vi "SetGet EMIccdGainControlMode.vi"(6 "wait for reply (T)":bool=TRUE, 7 "Broadcast":bool, 8 "error in (no error)":errorcluster, 9 "SetOrGet":T3, 10 "EMIccdGainControlMode":T2) -> (0 "error out":errorcluster, 1 "timed out?":bool, 2 "Reply Payload":T1)   [LabVIEW 2019, in "Camera.lvlib"]
doc: "_____\nCreated using Delacor QMH Event Scripter 5.0.0.112."
uses:
  Camera.lvlib
  picam32_LabView_SDK/PICam_lib/types/PicamEMIccdGainControlMode.ctl
  Utility/Types/SetOrGet.ctl
  SetGet EMIccdGainControlMode (Reply Payload)--cluster.ctl
  SetGet EMIccdGainControlMode Argument--cluster.ctl
  picam32_LabView_SDK/PICam_lib/PICam.lvlib
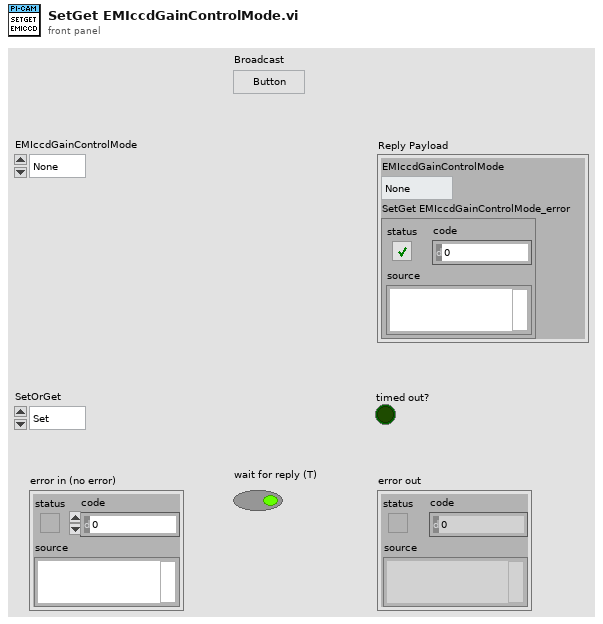
[diagram p1: front panel]
types:
  T1 = typedef "Camera.lvlib/SetGet EMIccdGainControlMode (Reply Payload)--cluster.ctl" = cluster{"EMIccdGainControlMode":T2, "SetGet EMIccdGainControlMode_error":errorcluster}
  T2 = typedef "PICam.lvlib/PicamEMIccdGainControlMode.ctl" = enum16{"None", "Optimal", "Manual"}
  T3 = typedef "SetOrGet.ctl" = enum16{"Set", "Get"}
  T4 = typedef "Camera.lvlib/SetGet EMIccdGainControlMode Argument--cluster.ctl" = cluster{"EMIccdGainControlMode":T2, "SetOrGet":T3, "Broadcast":bool, "Wait Notifier":refnum<notifier>, "wait for reply":bool}
  T5 = typedef "Camera.lvlib/Request Events--cluster.ctl" = cluster{"Stop Module":refnum<user-event>, "Show Panel":refnum<user-event>, "Hide Panel":refnum<user-event>, "Get Module Execution Status":refnum<user-event>, "Show Diagram":refnum<user-event>, "Get Image":refnum<user-event>, "Set Accumulations":refnum<user-event>, "Set ROI":refnum<user-event>, "Acquire Image":refnum<user-event>, "Acquire Continuously":refnum<user-event>, "Acquisition Done":refnum<user-event>, "Get Module Data":refnum<user-event>, "Stop Acquisition":refnum<user-event>, "Set GatingMode":refnum<user-event>, "Get GatingMode":refnum<user-event>, "Set RepetitiveGate":refnum<user-event>, "Get RepetitiveGate":refnum<user-event>, "Get IntensifierStatus":refnum<user-event>, "EnableIntensifier":refnum<user-event>, "Set IntensifierGain":refnum<user-event>, "Get IntensifierGain":refnum<user-event>, "SetGet EMIccdGainControlMode":refnum<user-event>, "SetGet EMIccdGain":refnum<user-event>, "SetGet FloatingPoint Parameter":refnum<user-event>, "SetGet Integer Parameter":refnum<user-event>, "SetGet LargeInteger Parameter":refnum<user-event>, "SetGet Pulse Parameter":refnum<user-event>}
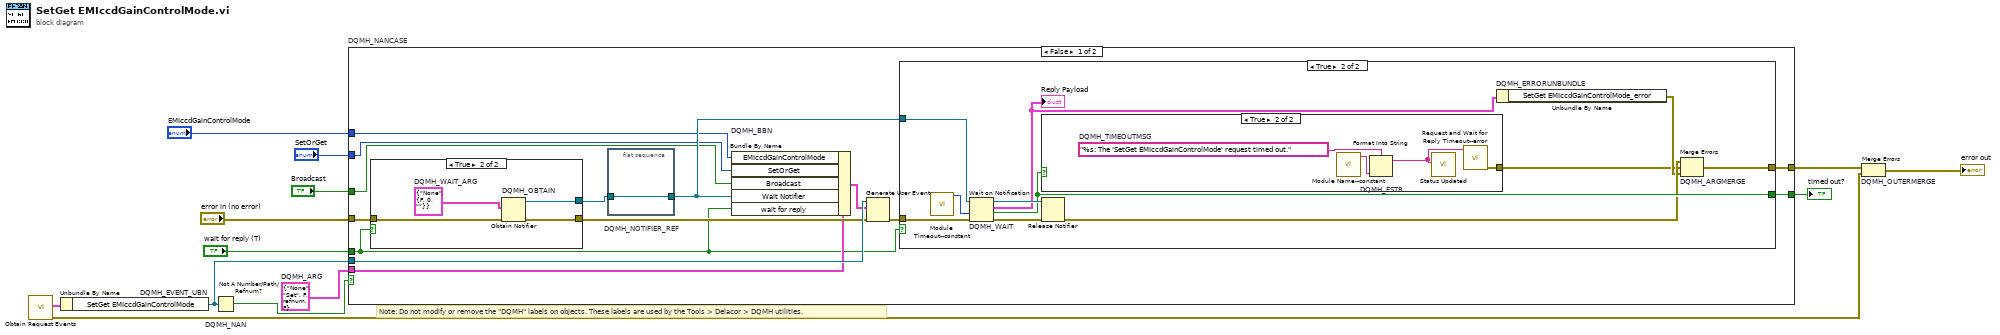
[diagram p0: block diagram]
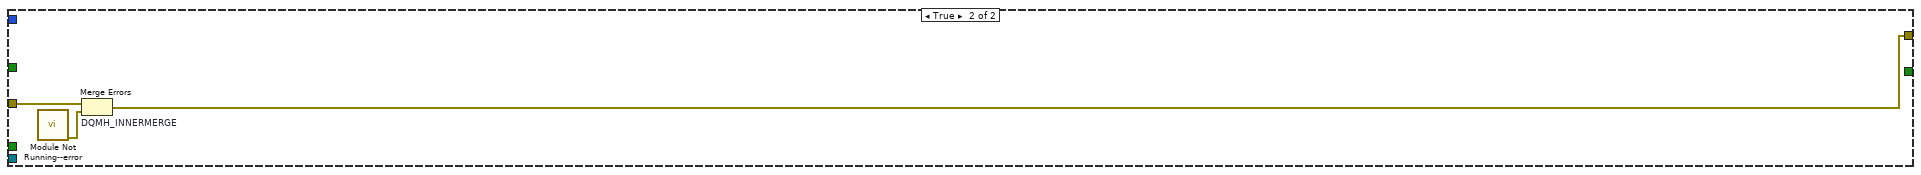
[diagram p5: hidden frame]
diagram:
  w7 = T4 {"EMIccdGainControlMode"=enum."None", "SetOrGet"=enum."Set", "Broadcast"=FALSE, "Wait Notifier"=refnum, "wait for reply"=FALSE}  # DQMH_ARG
  # "Note: Do not modify or remove the \"DQMH\" labels on objects. These labels are used by the Tools > Delacor > DQMH utilities."
  n1 = call "Obtain Request Events.vi"() -> ("error out"=w2:errorcluster, "Camera Request Events"=w1:T5)  [unwired: 10 in]
  n2 = Unbundle By Name "DQMH_EVENT_UBN"(w1) -> ("SetGet EMIccdGainControlMode"=w11:refnum<user-event>)
  n3 = Not A Number/Path/Refnum? "DQMH_NAN"(number/path/refnum=w11) -> (NaN/Path/Refnum?=w10:bool)
  n4 = case "DQMH_NANCASE" shown="False" w10 {
    tunnel: "error in (no error)" -> [w27 w52]
    tunnel: w11 -> [w25 _]
    tunnel: [w22 w51] -> w8
    tunnel: [w23 _] -> w9
    tunnel: w7 -> [w18 _]
    tunnel: "EMIccdGainControlMode" -> [w17 _]
    tunnel: "SetOrGet" -> [w16 _]
    tunnel: "Broadcast" -> [w15 _]
    tunnel: "wait for reply (T)" -> [w14 _]
    frame False {
      n5 = case shown="True" w14 {
        tunnel: w27 -> [w45 w49]
        tunnel: [w45 w48] -> w24
        tunnel: [_ w46] -> w20
        frame False {
        }
        frame True {
          w47 = T1 {"EMIccdGainControlMode"=enum."None", "SetGet EMIccdGainControlMode_error"={"status"=FALSE, "code"=0, "source"=""}}  # DQMH_WAIT_ARG
          n6 = Obtain Notifier "DQMH_OBTAIN"(notification data type=w47, error in (no error)=w49) -> (notifier out=w46:refnum<notifier>, error out=w48:errorcluster)  [unwired: 2 in, 1 out]
        }
      }
      n7 = flat-sequence "DQMH_NOTIFIER_REF" {
        tunnel: w20 -> [w28]
        tunnel: [w28] -> w19
        frame #0 {
        }
      }
      n8 = Bundle By Name "DQMH_BBN"(cluster=w18, "EMIccdGainControlMode"=w17, "SetOrGet"=w16, "Broadcast"=w15, "Wait Notifier"=w19, "wait for reply"=w14) -> (w21:T4)
      n9 = Generate User Event(user event=w25, event data cluster=w21, error in=w24) -> (error out=w26:errorcluster)  [unwired: 1 in, 1 out]
      n10 = case shown="True" w14 {
        tunnel: w26 -> [w29 w40]
        tunnel: w19 -> [_ w39]
        tunnel: [_ w37] -> w23
        tunnel: [w29 w36] -> w22
        frame False {
        }
        frame True {
          n11 = call "Module Timeout--constant.vi"() -> ("Module Timeout"=w30:i32)  [unwired: 11 in]
          n12 = Wait on Notification "DQMH_WAIT"(notifier=w39, timeout in ms (-1)=w30, error in (no error)=w40) -> (notifier out=w38:refnum<notifier>, notification=w35:T1, timed out?=w37:bool, error out=w34:errorcluster)  [unwired: 1 in]
          "Reply Payload" <- w35
          n13 = case shown="True" w37 {
            tunnel: [_ w42] -> w31
            frame False {
            }
            frame True {
              w44 = "%s: The 'SetGet EMIccdGainControlMode' request timed out."  # DQMH_TIMEOUTMSG
              n14 = call "Module Name--constant.vi"() -> ("Module Name"=w41:string)  [unwired: 11 in]
              n15 = Format Into String "DQMH_FSTR"(format string=w44, w41) -> (resulting string=w43:string)  [unwired: 2 in, 1 out]
              n16 = call "Status Updated.vi"("Status"=w43) -> ()  [unwired: 10 in, 1 out]
              n17 = call "Request and Wait for Reply Timeout--error.vi"("Error Message"=w43) -> ("error out"=w42:errorcluster)  [unwired: 10 in]
            }
          }
          n18 = Release Notifier(notifier=w38, error in (no error)=w34) -> (error out=w33:errorcluster)  [unwired: 1 in, 2 out]
          n19 = Unbundle By Name "DQMH_ERRORUNBUNDLE"(w35) -> ("SetGet EMIccdGainControlMode_error"=w32:errorcluster)
          n20 = Merge Errors "DQMH_ARGMERGE"(w33, w31, w32) -> (w36:errorcluster)
        }
      }
    }
    frame True {
      n21 = call "Module Not Running--error.vi"() -> ("error out"=w50:errorcluster)  [unwired: 11 in]
      n22 = Merge Errors "DQMH_INNERMERGE"(w52, w50) -> (w51:errorcluster)
    }
  }
  "timed out?" <- w9
  n23 = Merge Errors "DQMH_OUTERMERGE"(w8, w2) -> (→"error out":errorcluster)
